vi "Switchboard.vi"(11 "Sensor type":enum16{"6''", "8''", "One channel"}(ring)) -> (3 "Output config":i32[](array[numeric]))   [LabVIEW 2015]
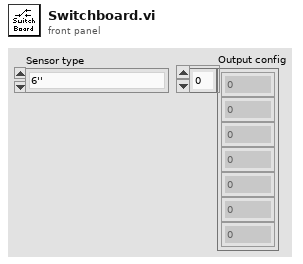
[diagram p1: front panel]
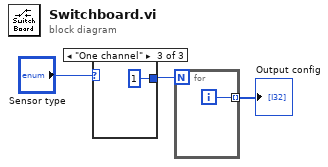
[diagram p0: block diagram]
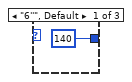
[diagram p2: hidden frame]
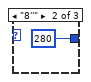
[diagram p3: hidden frame]
diagram:
  n1 = case shown="\"One channel\"" "Sensor type" {
    tunnel: [140 280 1] -> w1
    frame "6''", Default {
    }
    frame "8''" {
    }
    frame "One channel" {
    }
  }
  n2 = for {
    N: w1 -> [_]
    tunnel: [w7] -> w3 mode=indexing
    i -> [w7]
  }
  "Output config" <- w3
